vi "Power Of X - RM,I.vi"(1 "Real Matrix A":T1, 2 "Power n":i32) -> (0 "A^n":T1)   [LabVIEW 2014, in "NI_Matrix.lvlib"]
doc: "Computes the nth power of the input matrix."
uses:
  NI_Matrix.lvlib
  RealMatrix.ctl
  Real Matrix Power.vi
  NI_AALBase.lvlib
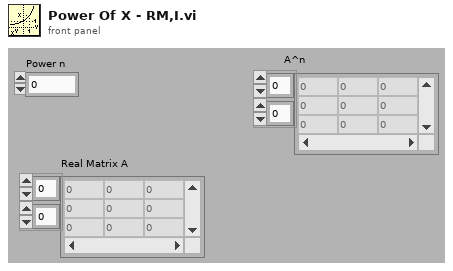
[diagram p1: front panel]
types:
  T1 = typedef "NI_Matrix.lvlib/RealMatrix.ctl" = dbl[][]
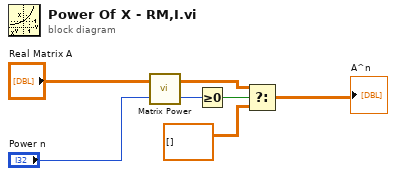
[diagram p0: block diagram]
diagram:
  n1 = call-poly "Matrix Power.vi"("n"="Power n", "Input Matrix"="Real Matrix A") -> ("error"=w2:i32, "Matrix Power"=w1:T1)
  n2 = Greater Or Equal To 0?(x=w2) -> (x >= 0?=w7:bool)
  n3 = Select(t=w1, s=w7, f=T1 [] ("A * c")) -> (s? t:f=→"A^n":T1)
